vi "Vision Research Phantom Series PhCon PhGetBitDepths.vi"(0 "CN in":u32=1, 5 "Error In (no error)":errorcluster) -> (14 "CN out":u32=1, 16 "pCnt":u32=1, 17 "pVal":u32[](array[numeric]), 19 "Error Out":errorcluster)   [LabVIEW 2013, in "VRI.lvlib"]
doc: "PhCon.dll\n\nPhGetBitDepths\nHRESULT PhGetBitDepths(UINT CN, PUINT pCnt, PUINT pVal)\n\nParameters Description\nCN (in) Camera number.\npCnt (out) Count of values of the result.\npVal (out) Provides a list of the possible pixel bit depths when\n recording in the camera FBM. Example: the Phantom\n v9.1 camera can record at 8, 10, 12, 14, 16 bits per\n pixel. Larger bit depths may provide better image or\n better sensitivity but decrease the number of images\n that can be recorded.\n The bit depths are stored in the array in increasing \n order."
uses:
  VRI.lvlib
  Phantom DLLs/PhCon.Dll
panel:
  # "For instructions on the use of this VI, press Ctrl+H to display the help window and move the mouse over the icon, controls, and indicators"
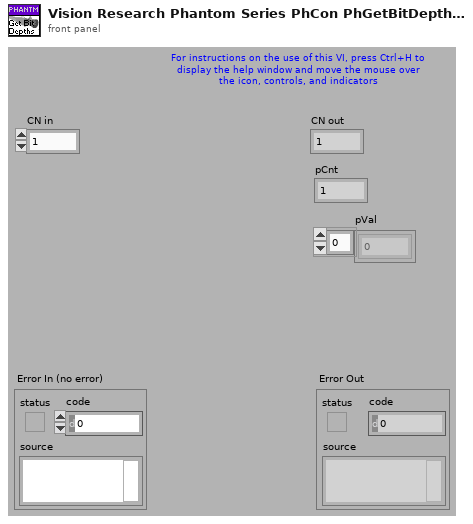
[diagram p1: front panel]
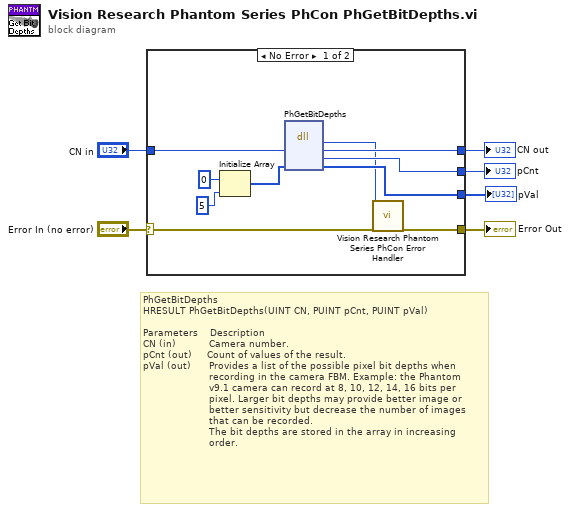
[diagram p0: block diagram]
diagram:
  # "PhGetBitDepths\nHRESULT PhGetBitDepths(UINT CN, PUINT pCnt, PUINT pVal)\n\nParameters    Description\nCN (in)           Camera number.\npCnt (out)     Count of values of the result.\npVal (out)      Provides a list of the possible pixel bit depths when\n                      recording in the camera FBM. Example: the Phantom\n                      v9.1 camera can record at 8, 10, 12, 14, 16 bits per\n                      pixel. Larger bit depths may provide better image or\n                      better sensitivity but decrease the number of images\n                      that can be recorded.\n                      The bit depths are stored in the array in increasing \n                      order."
  n1 = case shown="No Error" "Error In (no error)" {
    selector: "Error In (no error)" -> [w16 w18]
    tunnel: [w15 w18] -> w5
    tunnel: "CN in" -> [w14 w17]
    tunnel: [w13 w17] -> w3
    tunnel: [w12 _] -> w2
    tunnel: [w11 _] -> w1
    frame No Error {
      n2 = Initialize Array(u32 0 ("element"), 5 ("dimension size")) -> (w9:u32[])
      n3 = dll-call lib="C:/Projects/SDK/64-bit/Vision Research Phantom Series Labview Driver/Phantom DLLs/PhCon.dll" fn="PhGetBitDepths"("CN"=w14, "pVal"=w9) -> ("HRESULT"=w10:i32, "CN"=w13:u32, "pCnt"=w12:u32, "pVal"=w11:u32[])  [unwired: 3 in, 3 out]
      n4 = call "Vision Research Phantom Series PhCon Error Handler.vi"("ErrNo"=w10, "Error In (no error)"=w16) -> ("Error Out"=w15:errorcluster)  [unwired: 17 out]
    }
    frame Error {
    }
  }
  "Error Out" <- w5
  "CN out" <- w3
  "pCnt" <- w2
  "pVal" <- w1
